vi "Obliczenia_f_z_zakresu(SubVI).vi"(6 "Zakres":dbl, 9 "Szukana czêstotliwoœæ":dbl, 10 "magnitude":dbl[](array[numeric]), 11 "df":dbl) -> (1 "czêstotliwoœæ szukanej f":dbl, 2 "amplituda szukanej f":dbl format="%#_10g", 3 "probka":dbl)   [LabVIEW 2018]
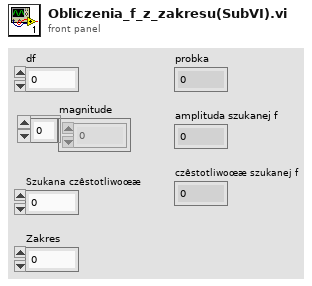
[diagram p1: front panel]
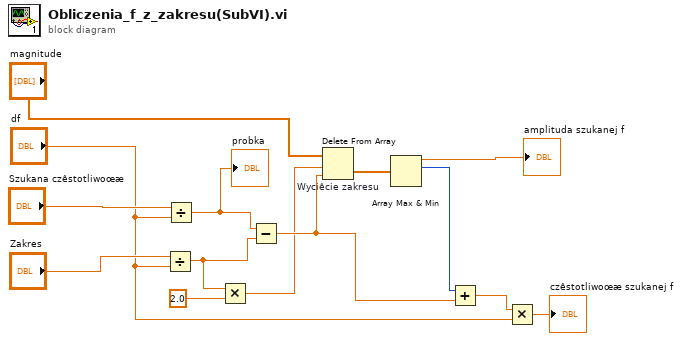
[diagram p0: block diagram]
diagram:
  n1 = Divide(x="Zakres", y="df") -> (x/y=w2:dbl)
  n2 = Divide(x="Szukana czêstotliwoœæ", y="df") -> (x/y=w1:dbl)
  "probka" <- w1
  n3 = Multiply(x=w2, y=2.0) -> (x*y=w4:dbl)
  n4 = Subtract(x=w1, y=w2) -> (x-y=w11:dbl)
  n5 = Delete From Array "Wyciêcie zakresu"(array="magnitude", length=w4, index=w11) -> (deleted portion=w14:dbl[])  [unwired: 1 out]
  n6 = Array Max & Min(array=w14) -> (max value=→"amplituda szukanej f":dbl, max index (indices)=w6:i32)  [unwired: 2 out]
  n7 = Add(x=w6, y=w11) -> (x+y=w7:dbl)
  n8 = Multiply(x=w7, y="df") -> (x*y=→"czêstotliwoœæ szukanej f":dbl)
